vi "Write Current.vi"(8 "error in":errorcluster, 10 "Current":dbl, 11 "69X_79X in":refnum<class "6972A.lvclass">) -> (0 "error out":errorcluster, 3 "69X_79X out":refnum<class "6972A.lvclass">)   [LabVIEW 2019, in "6972A.lvlib" / "6972A.lvclass"]
uses:
  Library/6972A.lvclass
  C:/Users/Public/Documents/Development/builds/Instruments/PowerSupply.lvlibp/Library/PowerSupply.lvclass
  Library/6972A.lvclass/6972A.ctl
  Read Local Resource.vi
  builds/Instruments/PowerSupply.lvlibp/Library/PowerSupply.lvclass
  <instrlib>/Agilent N6900 N7900 Series/Agilent N6900 N7900 Series.lvlib
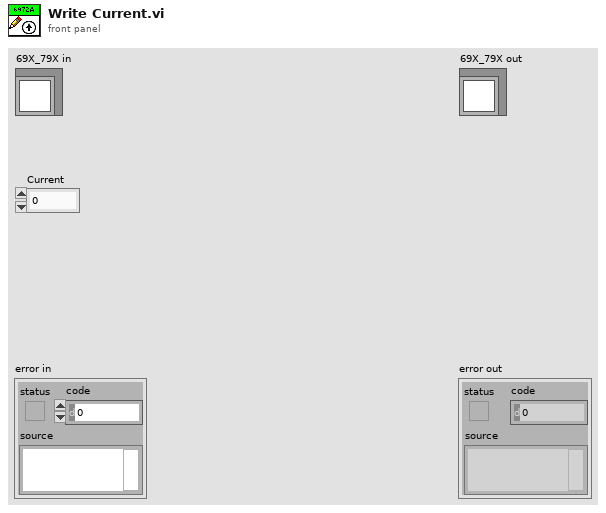
[diagram p1: front panel]
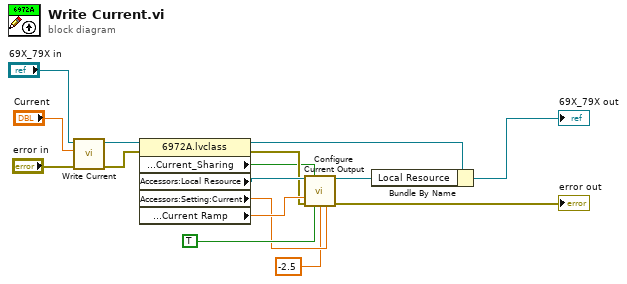
[diagram p0: block diagram]
diagram:
  n1 = call-parent "Write Current.vi"("error in"="error in", "Current"="Current", "PowerSupply in"="69X_79X in") -> ("error out"=w11:errorcluster, "PowerSupply out"=w13:refnum<class "6972A.lvclass">)  [unwired: 7 in]
  n2 = property class="6972A.lvclass"(reference=w13, error in=w11) -> (reference out=w12:refnum<class "6972A.lvclass">, error out=w5:errorcluster, "Accessors:Setting:Current_Sharing"=w4:bool, "Accessors:Local Resource"=w10:refnum<visa-resource-name>, "Accessors:Setting:Current"=w2:dbl, "Accessors:Setting:Ramp:Current Ramp"=w9:dbl)
  n3 = call <instrlib>:"Configure Current Output.vi"("VISA resource name"=w10, "Enable Parallel Unit Sharing (False)"=w4, "Current Slew (Inf)"=w9, "error in (no error)"=w5, "Enable Voltage Priority (False)"=TRUE, "Voltage Priority Current Lower Limit (-2.50A)"=-2.5, "Voltage Priority Current Upper Limit (2.50A)"=w2) -> ("VISA resource name out"=w6:refnum<visa-resource-name>, "error out"=→"error out":errorcluster)  [unwired: 7 in]
  n4 = Bundle By Name(cluster=w12, "Local Resource"=w6) -> (→"69X_79X out":refnum<class "6972A.lvclass">)
